vi "E04_Tunel_SF.vi"() -> ()   [LabVIEW 2026]
panel:
  out "SF0 3":i32
  out "SF0 2":i32
  out "Arreglo (indexado)":i32[](array[numeric])
  out "Ultimo valor":i32
  out "SF0":i32
  out "Shift register":i32
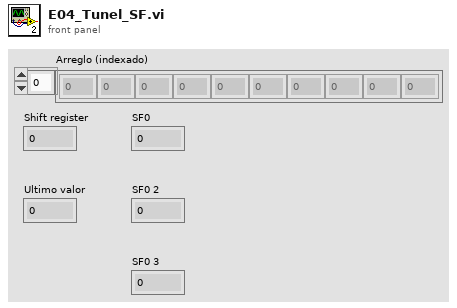
[diagram p1: front panel]
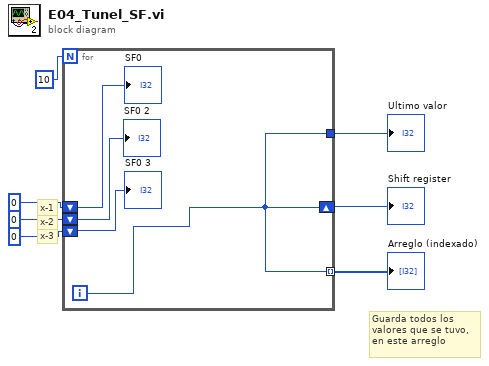
[diagram p0: block diagram]
diagram:
  # "Guarda todos los\nvalores que se tuvo, \nen este arreglo"
  # "x-3"
  # "x-2"
  # "x-1"
  n1 = for {
    N: 10 -> [_]
    shift-right: [w10] -> w6
    shift-left: 0 -> [w11]
    tunnel: [w10] -> w5
    tunnel: [w10] -> w4 mode=indexing
    shift-left: 0 -> [w9]
    shift-left: 0 -> [w8]
    i -> [w10]
    "SF0" <- w11
    "SF0 2" <- w9
    "SF0 3" <- w8
  }
  "Shift register" <- w6
  "Ultimo valor" <- w5
  "Arreglo (indexado)" <- w4
